vi "Get Power Supply Measurement.vi"(0 "Power Supply Address":refnum<visa-resource-name>, 1 "Power Supply Model":T1=enum."Keithley 24XX", 2 "error in":errorcluster) -> (3 "VISA resource name out":refnum<visa-resource-name>, 4 "Voltage Output":dbl, 5 "Current Output":dbl, 6 "error out":errorcluster)   [LabVIEW 2020]
uses:
  Typedefs/Power Supply Models.ctl
  <instrlib>/Keithley 24XX/Keithley 24XX.lvlib
  <instrlib>/Agilent 6XXX Series/Agilent 6XXX Series.lvlib
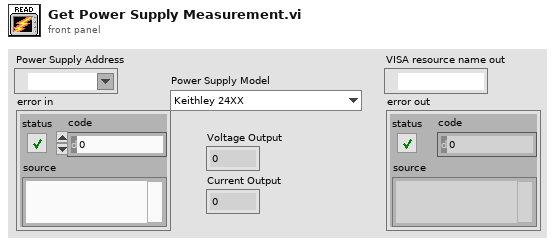
[diagram p1: front panel]
types:
  T1 = typedef "Power Supply Models.ctl" = enum16{"Keithley 248", "Keithley 237", "Keithley 24XX", "HP/Agilent 6XXX"}
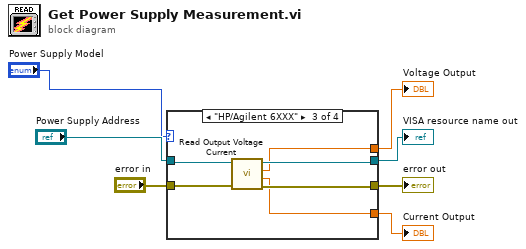
[diagram p0: block diagram]
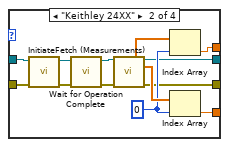
[diagram p3: hidden frame]
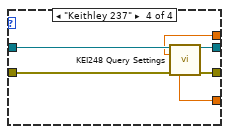
[diagram p4: hidden frame]
diagram:
  n1 = case shown="\"HP/Agilent 6XXX\"" "Power Supply Model" {
    tunnel: "Power Supply Address" -> [w8 w17 w27 w34]
    tunnel: [_ w13 w23 w33] -> w5
    tunnel: [_ w12 w24 w32] -> w4
    tunnel: [w9 w11 w25 w31] -> w2
    tunnel: "error in" -> [w9 w18 w28 w30]
    tunnel: [w8 w10 w26 w29] -> w3
    frame "Keithley 248", Default {
    }
    frame "Keithley 24XX" {
      w14 = 0
      n2 = call <instrlib>:"Initiate.vi"("error in (no error)"=w18, "VISA resource name"=w17) -> ("error out"=w21:errorcluster, "VISA resource name out"=w22:refnum<visa-resource-name>)  [unwired: 8 in]
      n3 = call <instrlib>:"Wait for Operation Complete.vi"("error in (no error)"=w21, "VISA resource name"=w22) -> ("error out"=w20:errorcluster, "VISA resource name out"=w19:refnum<visa-resource-name>)  [unwired: 8 in]
      n4 = call <instrlib>:"Fetch (Measurements).vi"("VISA resource name"=w19, "error in (no error)"=w20) -> ("Voltage"=w16:sgl[], "VISA resource name out"=w10:refnum<visa-resource-name>, "Current"=w15:sgl[], "error out"=w11:errorcluster)  [unwired: 7 in, 3 out]
      n5 = Index Array(array=w16, index=w14) -> (element=w13:sgl)
      n6 = Index Array(array=w15, index=w14) -> (element=w12:sgl)
    }
    frame "HP/Agilent 6XXX" {
      n7 = call <instrlib>:"Read Output Voltage Current.vi"("error in (no error)"=w28, "VISA resource name"=w27) -> ("error out"=w25:errorcluster, "output current"=w24:dbl, "output voltage"=w23:dbl, "VISA resource name out"=w26:refnum<visa-resource-name>)  [unwired: 6 in]
    }
    frame "Keithley 237" {
      n8 = call "KEI248 Query Settings"("VISA resource name"=w34, "error in (no error)"=w30) -> ("VISA resource name out"=w29:refnum<visa-resource-name>, "Voltage Output"=w33:dbl, "Current Output"=w32:dbl, "error out"=w31:errorcluster)  [unwired: 3 in, 7 out]
    }
  }
  "Voltage Output" <- w5
  "Current Output" <- w4
  "VISA resource name out" <- w3
  "error out" <- w2
